vi "Manage Keep Alive.vi"(8 "error in (no error)":errorcluster, 9 "Reset Keepalive":bool, 10 "Keep Alive (sec)":u16, 11 "SubscriberQ":refnum<queue>) -> (0 "error out":errorcluster, 4 "Elapsed Time (s)":dbl)   [LabVIEW 2018]
uses:
  Message Queue/Message Cluster.ctl
  Message Queue/Enqueue Message (Single).vi
  Message Queue/Message Queue.lvlib
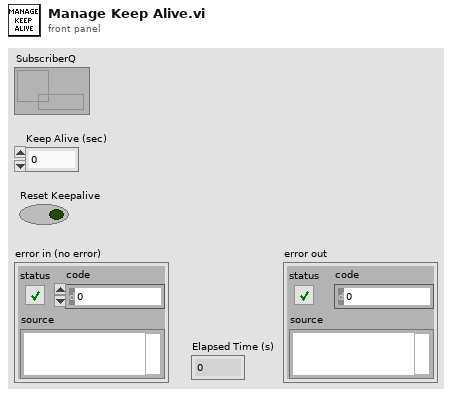
[diagram p1: front panel]
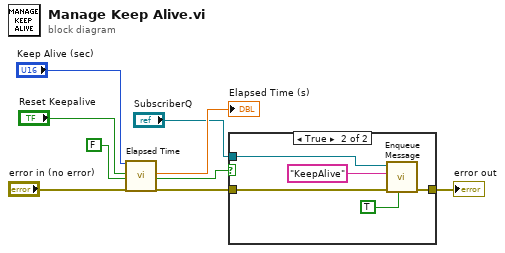
[diagram p0: block diagram]
diagram:
  n1 = call "Elapsed Time"("Time Target (s)"="Keep Alive (sec)", "Reset"="Reset Keepalive", "Auto Reset"=FALSE, "error in (no error)"="error in (no error)") -> ("Elapsed Time (s)"=→"Elapsed Time (s)":dbl, "Time has Elapsed"=w2:bool, "error out"=w8:errorcluster)  [unwired: 8 in, 5 out]
  n2 = case shown="True" w2 {
    tunnel: "SubscriberQ" -> [_ w15]
    tunnel: w8 -> [w10 w14]
    tunnel: [w10 w11] -> w9
    frame False {
    }
    frame True {
      n3 = call-poly "Enqueue Message.vi"("Priority Message? (F)"=TRUE, "error in (no error)"=w14, "Message"="KeepAlive", "Message Queue"=w15) -> ("error out"=w11:errorcluster)  [unwired: 6 in, 1 out]
    }
  }
  "error out" <- w9
